vi "Read User Names and Passwords.vi"(10 "Base Path":path) -> (1 "Passwords":string[](array[string]), 2 "access levels":i32[](array[numeric]), 3 "User Names":string[](array[string]))   [LabVIEW 2014]
uses:
  <vilib>/Utility/config.llb/Read Key (String).vi
  <vilib>/Utility/config.llb/Write Key (I32).vi
  <vilib>/Utility/config.llb/Read Key (I32).vi
  <vilib>/Utility/config.llb/NI_LVConfig.lvlib
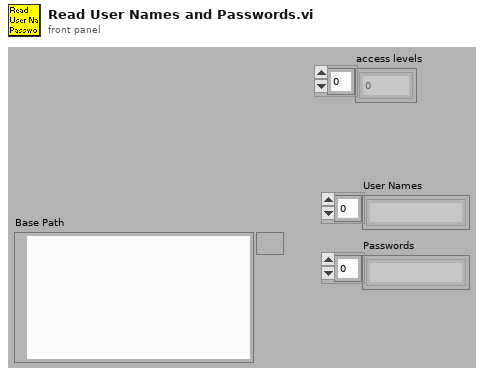
[diagram p1: front panel]
types:
  T1 = typedef "NI_LVConfig.lvlib/Config Data RefNum.ctl" = refnum<k1>
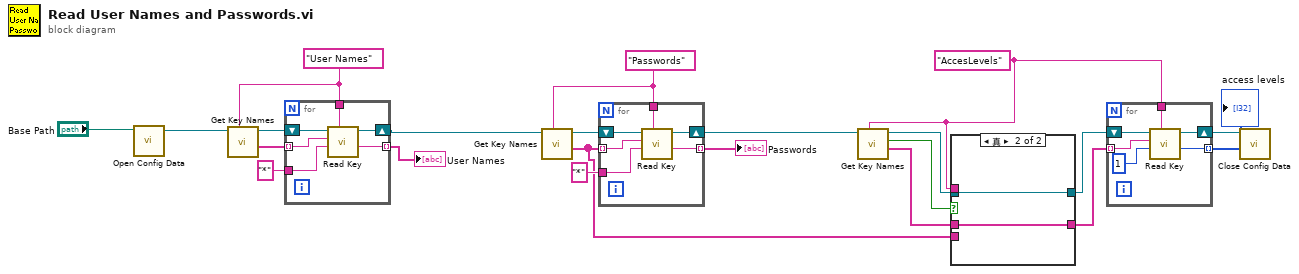
[diagram p0: block diagram]
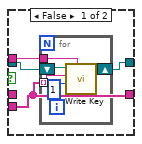
[diagram p2: hidden frame]
diagram:
  w2 = "AccesLevels" ("section")
  w13 = "Passwords" ("section")
  w21 = "User Names" ("section")
  n1 = call <vilib>:"Open Config Data.vi"("configuration file path"="Base Path") -> ("refnum"=w22:T1)  [unwired: 8 in, 2 out]
  n2 = call <vilib>:"Get Key Names.vi"("section"=w21, "refnum"=w22) -> ("key names"=w19:string[], "refnum out"=w20:T1)  [unwired: 6 in, 2 out]
  n3 = for {
    tunnel: w21 -> [w28]
    tunnel: w19 -> [w26] mode=indexing
    tunnel: "*" -> [w25]
    tunnel: [w24] -> w17 mode=indexing
    shift-right: [w23] -> w12
    shift-left: w20 -> [w27]
    n4 = call-poly <vilib>:"Read Key.vi"("section"=w28, "default value"=w25, "key"=w26, "refnum"=w27) -> ("value"=w24:string, "refnum out"=w23:T1)  [unwired: 4 in, 2 out]
  }
  "User Names" <- w17
  n5 = call <vilib>:"Get Key Names.vi"("section"=w13, "refnum"=w12) -> ("key names"=w1:string[], "refnum out"=w14:T1)  [unwired: 6 in, 2 out]
  n6 = for {
    tunnel: w13 -> [w34]
    tunnel: w1 -> [w32] mode=indexing
    tunnel: "*" -> [w31]
    tunnel: [w30] -> w16 mode=indexing
    shift-right: [w29] -> w10
    shift-left: w14 -> [w33]
    n7 = call-poly <vilib>:"Read Key.vi"("section"=w34, "default value"=w31, "key"=w32, "refnum"=w33) -> ("value"=w30:string, "refnum out"=w29:T1)  [unwired: 4 in, 2 out]
  }
  "Passwords" <- w16
  n8 = call <vilib>:"Get Key Names.vi"("section"=w2, "refnum"=w10) -> ("key names"=w4:string[], "section exists?"=w7:bool, "refnum out"=w6:T1)  [unwired: 6 in, 1 out]
  n9 = case shown="真" w7 {
    tunnel: [w38 w45] -> w5
    tunnel: w6 -> [w37 w45]
    tunnel: [w35 w44] -> w3
    tunnel: w4 -> [_ w44]
    tunnel: w2 -> [w36 _]
    tunnel: w1 -> [w35 _]
    frame False {
      n10 = for {
        shift-right: [w43] -> w38
        shift-left: w37 -> [w42]
        tunnel: w36 -> [w41]
        tunnel: w35 -> [w40] mode=indexing
        n11 = call-poly <vilib>:"Write Key.vi"("section"=w41, "value"=1, "key"=w40, "refnum"=w42) -> ("refnum out"=w43:T1)  [unwired: 5 in, 2 out]
      }
    }
    frame True {
    }
  }
  n12 = for {
    tunnel: w2 -> [w51]
    tunnel: w3 -> [w49] mode=indexing
    tunnel: [w48] -> w8 mode=indexing
    shift-right: [w47] -> w9
    shift-left: w5 -> [w50]
    n13 = call-poly <vilib>:"Read Key.vi"("section"=w51, "default value"=1, "key"=w49, "refnum"=w50) -> ("value"=w48:i32, "refnum out"=w47:T1)  [unwired: 4 in, 2 out]
  }
  "access levels" <- w8
  n14 = call <vilib>:"Close Config Data.vi"("refnum"=w9) -> ()  [unwired: 9 in, 2 out]
